vi "Connect.vi"(8 "Error In":errorcluster, 10 "Password":string, 11 "Username":string) -> (0 "Error Out":errorcluster, 3 "Nest Config":T1)   [LabVIEW 2013, in "LVH-Nest.lvlib"]
doc: "Establish a connection to the specified Nest devices."
uses:
  LVH-Nest.lvlib
  Private/Type Defs/Nest Config.ctl
  <vilib>/httpClient/ClientHandle.ctl
  Private/Type Defs/Session Data.ctl
  Private/Type Defs/Nest Error.ctl
  <vilib>/httpClient/POSTBuffer.vi
  <vilib>/httpClient/LabVIEWHTTPClient.lvlib
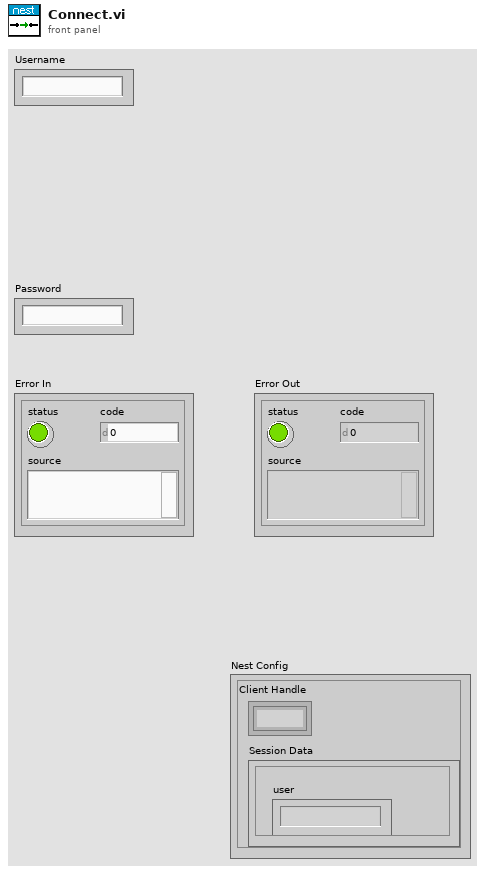
[diagram p1: front panel]
types:
  T1 = typedef "LVH-Nest.lvlib/Nest Config.ctl" = cluster{"Client Handle":T2, "Session Data":T3}
  T2 = typedef "LabVIEWHTTPClient.lvlib/ClientHandle.ctl" = refnum<k1>
  T3 = typedef "LVH-Nest.lvlib/Session Data.ctl" = cluster{"is_superuser":bool, "is_staff":bool, "urls":cluster{"transport_url":string, "rubyapi_url":string, "weather_url":string, "log_upload_url":string, "support_url":string}, "limits":cluster{"thermostats_per_structure":u32, "structures":u32, "thermostats":u32, "smoke_detectors":u32, "smoke_detectors_per_structure":u32}, "access_token":string, "userid":string, "expires_in":string, "email":string, "user":string, "language":string}
  T4 = typedef "LVH-Nest.lvlib/Nest Error.ctl" = enum16{"Unknown", "Auth", "Read", "Invalid Structure Name", "Invalid Device Name", "Set Temp"}
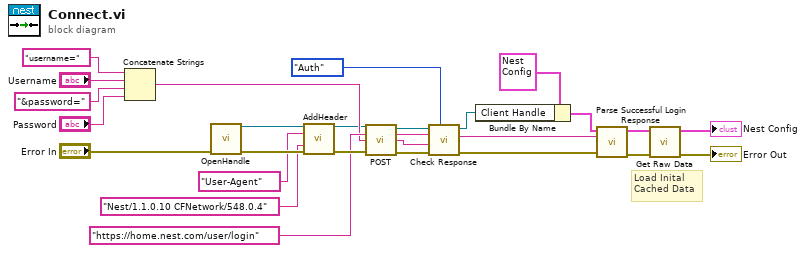
[diagram p0: block diagram]
diagram:
  # "Load Inital\nCached Data"
  n1 = Concatenate Strings("username=" ("string"), "Username", "&password=" ("string"), "Password") -> (w16:string)
  n2 = call <vilib>:"OpenHandle.vi"("error in (no error)"="Error In") -> ("client handle out"=w23:T2, "error out"=w21:errorcluster)  [unwired: 13 in]
  n3 = call <vilib>:"AddHeader.vi"("client handle"=w23, "header"="User-Agent", "value"="Nest/1.1.0.10 CFNetwork/548.0.4", "error in (no error)"=w21) -> ("client handle out"=w15:T2, "error out"=w18:errorcluster)  [unwired: 10 in]
  n4 = call-poly <vilib>:"POST.vi"("client handle"=w15, "url"="https://home.nest.com/user/login", "buffer"=w16, "error in (no error)"=w18) -> ("client handle out"=w13:T2, "headers"=w12:string, "body"=w8:string, "error out"=w14:errorcluster)  [unwired: 8 in]
  n5 = call "Check Response.vi"("Nest Error"=Nest_Error."Auth", "Error In"=w14, "Body"=w8, "Header"=w12, "Client Handle"=w13) -> ("Error Out"=w7:errorcluster, "Body"=w5:string, "Client Handle"=w9:T2)  [unwired: 3 in, 1 out]
  n6 = Bundle By Name(cluster=T1 {"Client Handle"=refnum, "Session Data"={"is_superuser"=FALSE, "is_staff"=FALSE, "urls"={"transport_url"="", "rubyapi_url"="", "weather_url"="", "log_upload_url"="", "support_url"=""}, "limits"={"thermostats_per_structure"=0, "structures"=0, "thermostats"=0, "smoke_detectors"=0, "smoke_detectors_per_structure"=0}, "access_token"="", "userid"="", "expires_in"="", "email"="", "user"="", "language"=""}} ("Nest Config"), "Client Handle"=w9) -> (w6:T1)
  n7 = call "Parse Successful Login Response.vi"("Error In"=w7, "Login Response"=w5, "Nest Config"=w6) -> ("Error Out"=w3:errorcluster, "Nest Config"=w4:T1)  [unwired: 7 in]
  n8 = call "Get Raw Data.vi"("Error In"=w3, "Nest Config"=w4) -> ("Error Out"=→"Error Out":errorcluster, "Nest Config"=→"Nest Config":T1)  [unwired: 7 in, 1 out]
